vi "rearrange booleans.vi"(11 "appended array":refnum<vi>[](array[refnum])) -> (3 "Numeric":u32)   [LabVIEW 2016]
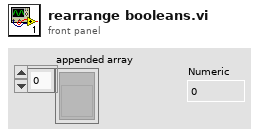
[diagram p1: front panel]
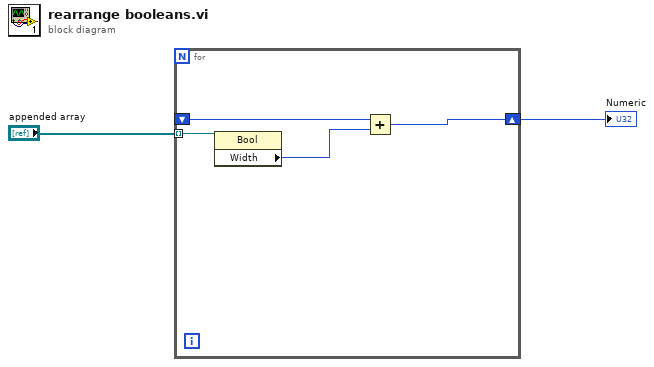
[diagram p0: block diagram]
diagram:
  n1 = for {
    tunnel: "appended array" -> [w6] mode=indexing
    shift-right: [w4] -> w1
    shift-left: _ -> [w3]
    n2 = property class="Bool"(reference=w6) -> ("Width"=w5:u32)  [unwired: 1 in, 2 out]
    n3 = Add(x=w3, y=w5) -> (x+y=w4:u32)
  }
  "Numeric" <- w1
